vi "sub_test.vi"(2 "Numeric 2":refnum<vi>, 8 "error in":errorcluster, 10 "stop":refnum<vi>) -> (0 "error out":errorcluster)   [LabVIEW 2018]
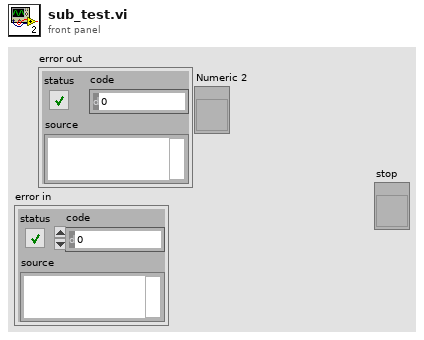
[diagram p1: front panel]
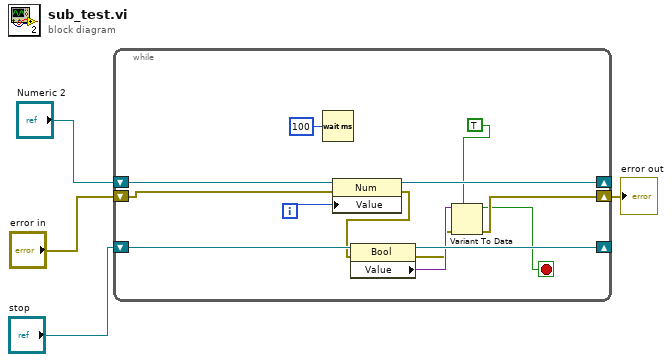
[diagram p0: block diagram]
diagram:
  n1 = while {
    shift-right: [w16] -> _
    shift-left: "Numeric 2" -> [w17]
    shift-right: [w7] -> w3
    shift-left: "error in" -> [w14]
    shift-right: [w12] -> _
    shift-left: "stop" -> [w11]
    i -> [w15]
    stop <- w5 stop-if-true
    n2 = Wait (ms)(milliseconds to wait=u32 100) -> ()  [unwired: 1 out]
    n3 = property class="Num"(reference=w17, error in=w14, "Value"=w15) -> (reference out=w16:refnum<vi>, error out=w9:errorcluster)
    n4 = property class="Bool"(reference=w11, error in=w9) -> (reference out=w12:refnum<vi>, error out=w8:errorcluster, "Value"=w10:variant)
    n5 = Variant To Data(error in=w8, type=TRUE, Variant=w10) -> (data=w5:bool, error out=w7:errorcluster)
  }
  "error out" <- w3
